vi "tstp_can_send_request.vi"(8 "error in (no error)":errorcluster, 9 "Data":u8[](array[numeric]), 10 "ADiagModuleIndex":i32, 11 "路径输入":path) -> (0 "error out":errorcluster, 2 "return":i32, 3 "路径输出":path)   [LabVIEW 2014]
doc: "根据物理地址Request ID发送数据"
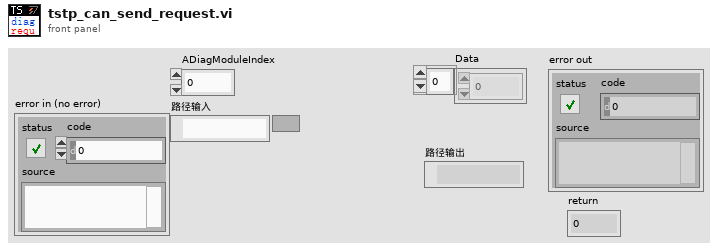
[diagram p1: front panel]
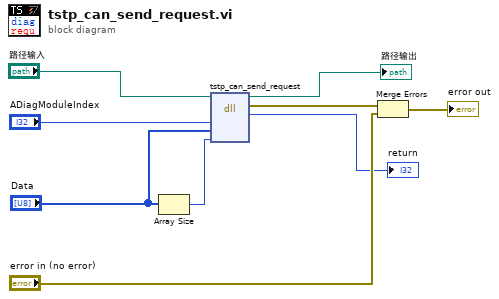
[diagram p0: block diagram]
diagram:
  n1 = Array Size(array="Data") -> (size(s)=w5:i32)
  n2 = dll-call lib="D:/Program Files (x86)/TOSUN/TSMaster/bin/TSMaster.dll" fn="tstp_can_send_request"(path in="路径输入", "ADiagModuleIndex"="ADiagModuleIndex", "AReqDataArray"="Data", "AReaDataSize"=w5) -> (path out=→"路径输出":path, error out=w9:errorcluster, "ACode"=→"return":i32)  [unwired: 5 in]
  n3 = Merge Errors(w9, "error in (no error)") -> (→"error out":errorcluster)
